vi "Add Mapping.vi"(8 "error in (no error)":errorcluster, 10 "scale index":i32, 11 "Scaling configuration in":refnum<class "Scaling configuration.lvclass">) -> (0 "error out":errorcluster, 3 "Scaling configuration out":refnum<class "Scaling configuration.lvclass">)   [LabVIEW 2013, in "Scaling configuration.lvclass"]
uses:
  Scaling configuration.lvclass
  <vilib>/NI/Tag Bus Module Framework/channel/TBM channel.lvclass
  controls/scale data types.ctl
  <vilib>/NI/Tag Bus Module Framework/channel/channel classification.ctl
  <vilib>/NI/Tag Bus/tag/Data Type.ctl
  <vilib>/NI/Tag Bus/tag/tag descriptor.lvclass
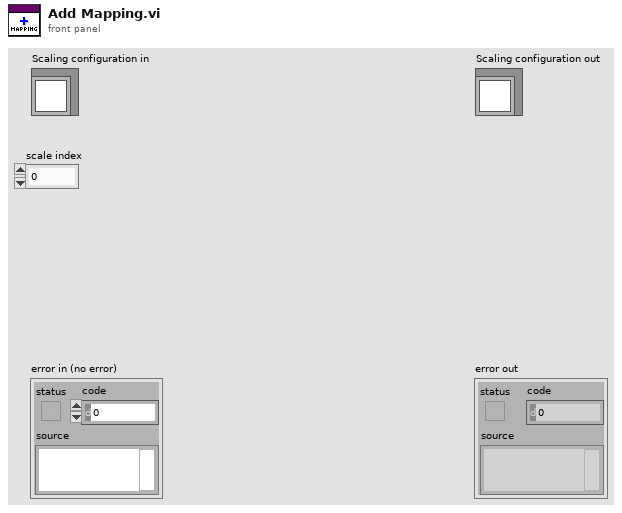
[diagram p1: front panel]
types:
  T1 = typedef "tag bus.lvlib/tag descriptor.lvclass/Data Type.ctl" = enum16{"Double", "Single", "I64", "I32", "I16", "I8", "U64", "U32", "U16", "U8", "Boolean", "String", "Array of Double", "Array of Single", "Array of I64", "Array of I32", "Array of I16", "Array of I8", "Array of U64", "Array of U32", "Array of U16", "Array of U8", "Array of Boolean", "Array of String"}
  T2 = typedef "TBM channel.lvclass/channel classification.ctl" = enum16{"input data", "output data", "processing parameter", "processing result"}
  T3 = typedef "Scaling configuration.lvclass/scale data types.ctl" = enum16{"Double", "Single", "I64", "I32", "I16", "I8", "U64", "U32", "U16", "U8"}
  T4 = cluster{"input channel":refnum<class "TBM channel.lvclass">, "output channel":refnum<class "TBM channel.lvclass">, "input data type":T3, "output data type":T3}
  T5 = cluster{"mappings":cluster{"input channel":refnum<class "TBM channel.lvclass">, "output channel":refnum<class "TBM channel.lvclass">, "input data type":T3, "output data type":T3}[], "name":string}[]
  T6 = cluster{"mappings":cluster{"input channel":refnum<class "TBM channel.lvclass">, "output channel":refnum<class "TBM channel.lvclass">, "input data type":T3, "output data type":T3}[], "name":string}
  T7 = cluster{"input channel":refnum<class "TBM channel.lvclass">, "output channel":refnum<class "TBM channel.lvclass">, "input data type":T3, "output data type":T3}[]
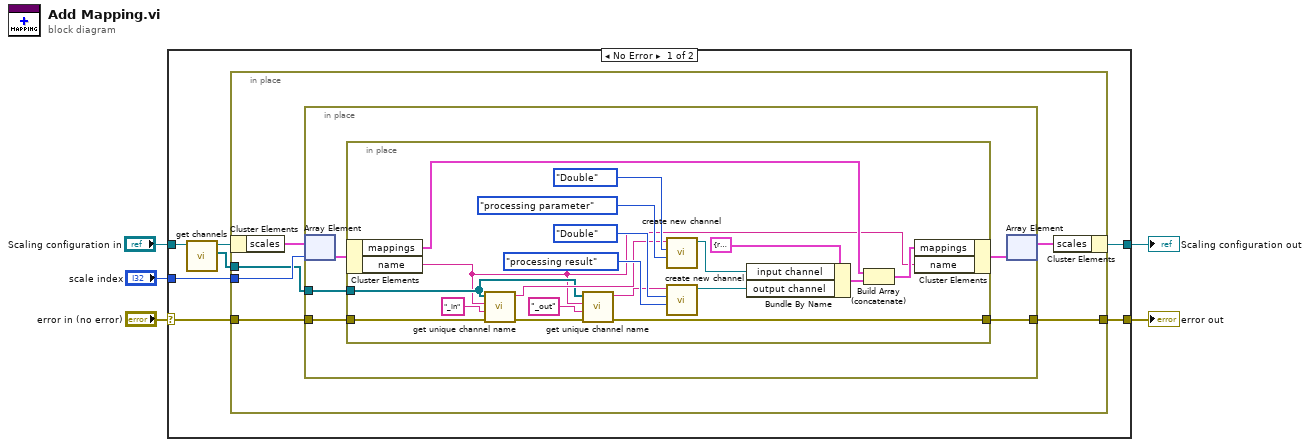
[diagram p0: block diagram]
diagram:
  n1 = case shown="No Error" "error in (no error)" {
    selector: "error in (no error)" -> [w10 w44]
    tunnel: [w9 w44] -> w4
    tunnel: [w12 w43] -> w2
    tunnel: "Scaling configuration in" -> [w8 w43]
    tunnel: "scale index" -> [w11 _]
    frame No Error {
      n2 = call-dynamic "get channels.vi"("Scaling configuration in"=w8) -> ("channels"=w6:refnum<class "TBM channel.lvclass">[], "Scaling configuration out"=w7:refnum<class "Scaling configuration.lvclass">)  [unwired: 9 in]
      n3 = in-place {
        in-place-border: w11 -> [w17]
        in-place-border: w10 -> [w15]
        in-place-border: [w14] -> w9
        in-place-border: w6 -> [w13]
        n4 = in-place-cluster #1(w7) -> ("scales"=w18:T5)
        n5 = in-place {
          in-place-border: w15 -> [w21]
          in-place-border: [w20] -> w14
          in-place-border: w13 -> [w19]
          n6 = in-place-array #2(w18, w17) -> (w23:T6)
          n7 = in-place {
            in-place-border: w21 -> [w29]
            in-place-border: [w28] -> w20
            in-place-border: w19 -> [w25]
            n8 = in-place-cluster #3(w23) -> ("mappings"=w42:T7, "name"=w24:string)
            n9 = call "get unique channel name.vi"("error in"=w29, "prefix"="_in", "scale name"=w24, "channels"=w25) -> ("error out"=w31:errorcluster, "name"=w32:string)  [unwired: 6 in]
            n10 = call "get unique channel name.vi"("error in"=w31, "prefix"="_out", "scale name"=w24, "channels"=w25) -> ("error out"=w28:errorcluster, "name"=w30:string)  [unwired: 6 in]
            n11 = call <vilib>:"create new channel.vi"("channel classification"=channel_classification."processing parameter", "data type"=Data_Type."Double", "channel name"=w32) -> ("channel"=w38:refnum<class "TBM channel.lvclass">)  [unwired: 8 in]
            n12 = call <vilib>:"create new channel.vi"("channel classification"=channel_classification."processing result", "data type"=Data_Type."Double", "channel name"=w30) -> ("channel"=w37:refnum<class "TBM channel.lvclass">)  [unwired: 8 in]
            n13 = Bundle By Name(cluster=T4 {"input channel"=refnum, "output channel"=refnum, "input data type"=enum."Double", "output data type"=enum."Double"} ("mapping"), "input channel"=w38, "output channel"=w37) -> (w39:T4)
            n14 = Build Array (concatenate)(w42, w39) -> (w41:T7)
            n15 = in-place-cluster #3("mappings"=w41, "name"=w24) -> (w22:T6)
          }
          n16 = in-place-array #2(w22) -> (w16:T5)  [unwired: 1 out]
        }
        n17 = in-place-cluster #1("scales"=w16) -> (w12:refnum<class "Scaling configuration.lvclass">)
      }
    }
    frame Error {
    }
  }
  "error out" <- w4
  "Scaling configuration out" <- w2
